vi "Builder Status.Get Build Durations.vi"(11 "Builder Status in":refnum<class "Builder Status.lvclass">) -> (2 "Build Durations":refnum<class "Memory.Pointer.U32.lvclass">, 3 "Builder Status out":refnum<class "Builder Status.lvclass">)   [LabVIEW 2016, in "DSF.Engine.lvlib" / "Builder Status.lvclass"]
uses:
  Builder Status.lvclass
  Submodules/Memory/Source/Classes/Standard Types/Memory.Pointer.U32.lvclass
  Builder Status.lvclass/Builder Status.ctl
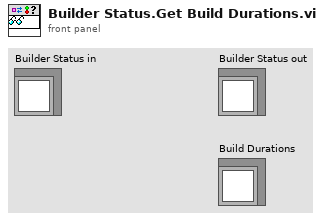
[diagram p1: front panel]
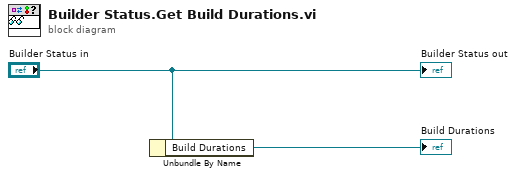
[diagram p0: block diagram]
diagram:
  n1 = Unbundle By Name("Builder Status in") -> ("Build Durations"=→"Build Durations":refnum<class "Memory.Pointer.U32.lvclass">)
  "Builder Status out" <- "Builder Status in"
